vi "niScope Configure Equalization Filter Coefficients.vi"(8 "error in":errorcluster, 9 "coefficients":dbl[](array[numeric]), 10 "channels":string="0", 11 "instrument handle":refnum<k15>) -> (0 "error out":errorcluster, 3 "instrument handle out":refnum<k15>)   [LabVIEW 2013]
doc: "Configures the custom coefficients for the equalization FIR filter on the device. This filter is designed to compensate the input signal for artifacts introduced to the signal outside of the digitizer. Because this filter is a generic FIR filter, any coefficients are valid. Coefficient values should be between +1 and -1."
uses:
  niScope_32.dll
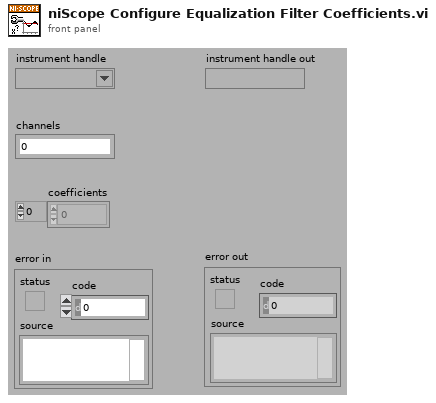
[diagram p1: front panel]
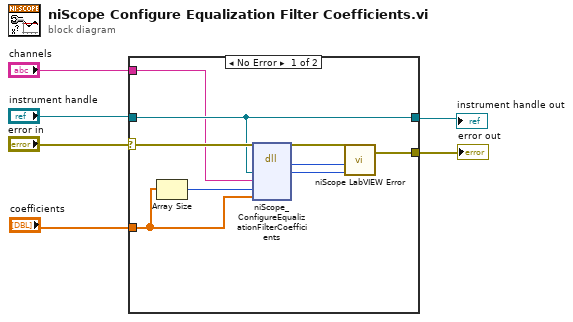
[diagram p0: block diagram]
diagram:
  n1 = case shown="No Error" "error in" {
    selector: "error in" -> [w11 w15]
    tunnel: [w12 w15] -> w6
    tunnel: "instrument handle" -> [w10 w16]
    tunnel: [w10 w16] -> w5
    tunnel: "coefficients" -> [w7 _]
    tunnel: "channels" -> [w9 _]
    frame No Error {
      n2 = Array Size(array=w7) -> (size(s)=w8:i32)
      n3 = dll-call lib="niScope_*.*" fn="niScope_ConfigureEqualizationFilterCoefficients"("instrument handle"=w10, "channel"=w9, "numCoefficients"=w8, "coefficients"=w7) -> ("status"=w14:i32, "instrument handle"=w13:u32)  [unwired: 6 in, 2 out]
      n4 = call <instrlib>:"niScope LabVIEW Error.vi"("instrument handle"=w13, "niScope error code (0)"=w14, "error in (no error)"=w11) -> ("error out"=w12:errorcluster)  [unwired: 2 in]
    }
    frame Error {
    }
  }
  "instrument handle out" <- w5
  "error out" <- w6
